vi "PhidgetLibraryVersion.vi"(8 "error in":errorcluster) -> (0 "error out":errorcluster, 2 "LibraryVersion":string caption="Library Version")   [LabVIEW 2012, in "Phidget Common.lvlib"]
doc: "${LibraryVersion:Header}"
uses:
  <instrlib>/Phidgets/Phidget Common/Phidget Common.lvlib
  <vilib>/Utility/importsl/GetValueByPointer/datatype.ctl
  <vilib>/Utility/importsl/GetValueByPointer/GetValueByPointer.xnode
  phidget22.dll
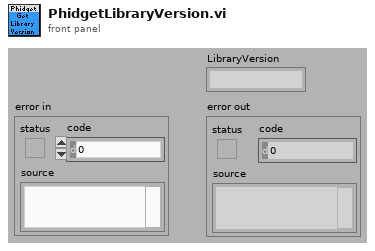
[diagram p1: front panel]
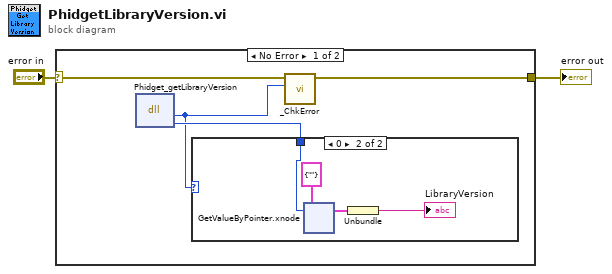
[diagram p0: block diagram]
diagram:
  n1 = case shown="No Error" "error in" {
    selector: "error in" -> [w6 w25]
    tunnel: [w5 w25] -> w1
    frame No Error {
      n2 = dll-call lib="phidget22.*" fn="Phidget_getLibraryVersion"() -> ("return type"=w3:i32, "DeviceLabel"=w4:u64)  [unwired: 4 in, 2 out]
      n3 = case shown="0" w3 {
        tunnel: w4 -> [_ w8]
        frame -1, Default {
        }
        frame 0 {
          n4 = xnode "GetValueByPointer.xnode"("Pointer"=w8, "InputType"=cluster{string} {""}) -> ("Output"=w9:cluster{string})  [unwired: 2 in, 1 out]
          n5 = Unbundle(w9) -> (→"LibraryVersion":string)
        }
      }
      n6 = call <instrlib>:"_ChkError.vi"("Return Code"=w3, "error in (no error)"=w6) -> ("error out"=w5:errorcluster)  [unwired: 9 in]
    }
    frame Error {
    }
  }
  "error out" <- w1
